vi "saltos.vi"(6 "Comienza Saltos":bool=TRUE, 8 "Nombre Imagen":string="foto", 9 "Path":path, 10 "Parametros de Saltos":T1={"Numero de Saltos"=6, "Paso del Salto (Hz)"=100.0, "Tiempo de estabilizacion (s)"=1.0, "Frequencia de estabilizacion (Hz)"=2000.0, "Tiempo de rampa ON (s)"=5.0, "Tiempo de rampa OFF (s)"=1.0}, 11 "Numero Ultimo Experimento":i32) -> (0 "Tomando Saltos":bool=TRUE, 1 "Estable":bool=TRUE, 2 "appended path":path, 3 "Freq Output":dbl, 4 "Numero Actual Experimento":i32, 5 "Captura Imagen":bool=TRUE)   [LabVIEW 2010]
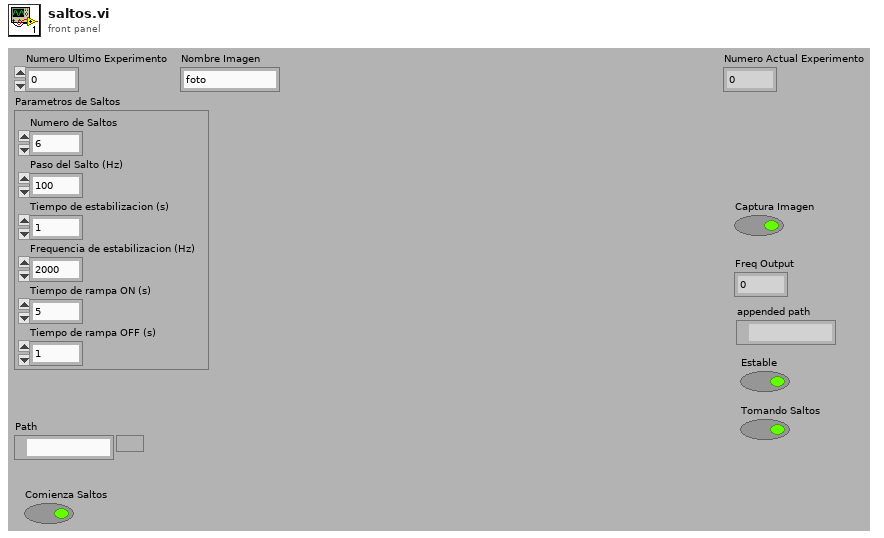
[diagram p1: front panel]
types:
  T1 = cluster{"Numero de Saltos":i32, "Paso del Salto (Hz)":dbl, "Tiempo de estabilizacion (s)":dbl, "Frequencia de estabilizacion (Hz)":dbl, "Tiempo de rampa ON (s)":dbl, "Tiempo de rampa OFF (s)":dbl}
  T2 = enum16{"Rampa ON", "Saltos", "Espera", "Toma Imagen", "Estable", "Rampa OFF", "Espera Estable"}
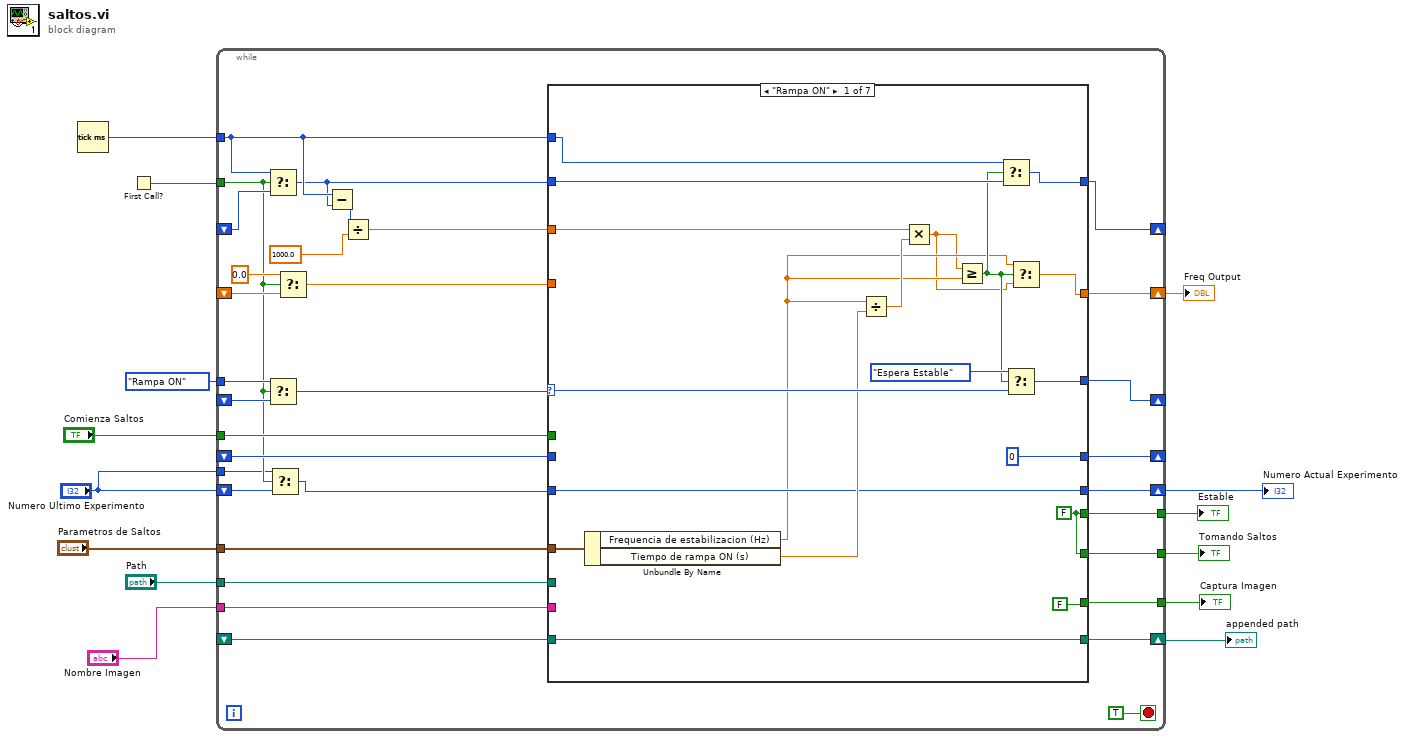
[diagram p0: block diagram]
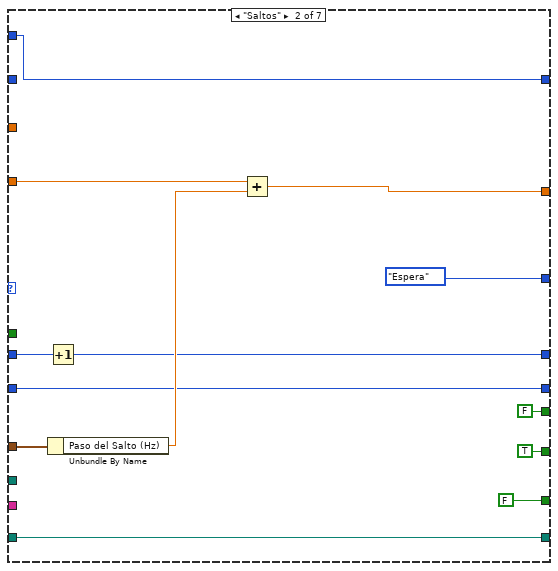
[diagram p2: hidden frame]
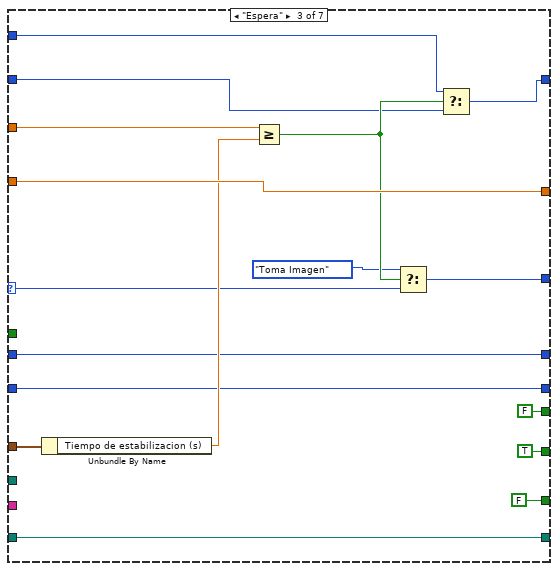
[diagram p3: hidden frame]
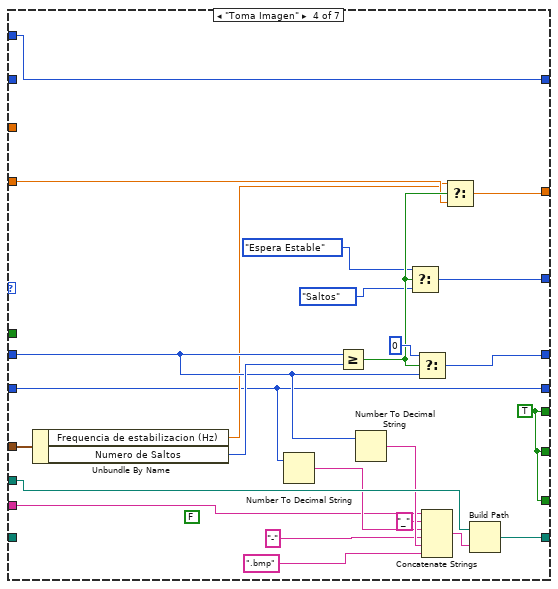
[diagram p4: hidden frame]
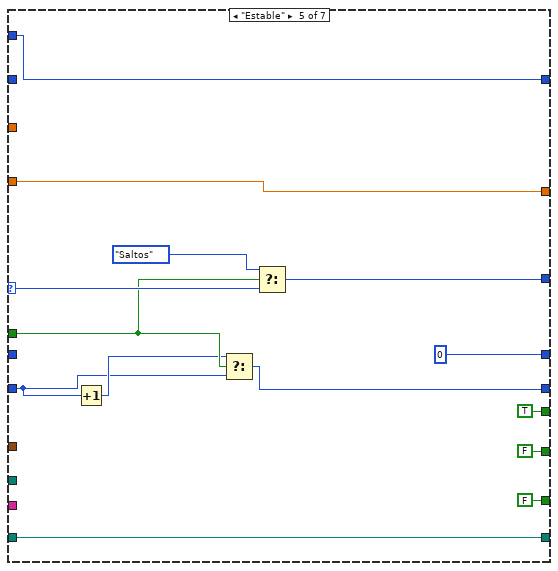
[diagram p5: hidden frame]
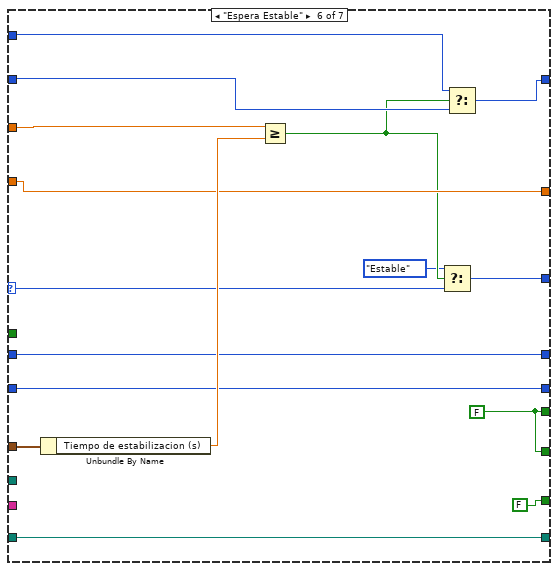
[diagram p6: hidden frame]
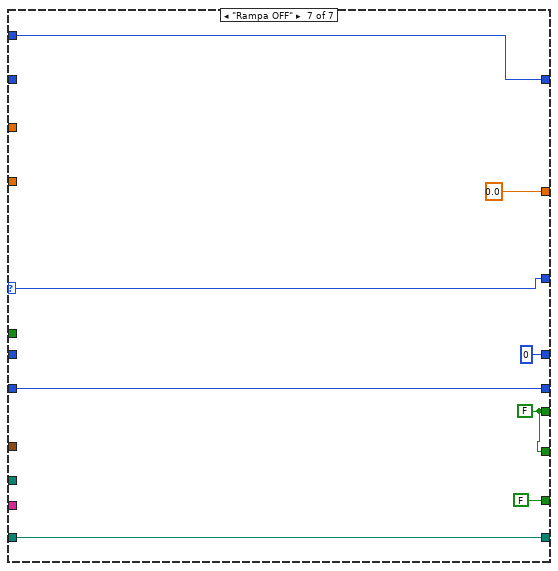
[diagram p7: hidden frame]
diagram:
  n1 = Tick Count (ms)() -> (millisecond timer value=w8:u32)
  n2 = First Call?() -> (First Call?: T/F=w14:bool)
  n3 = while {
    tunnel: w14 -> [w21]
    tunnel: w8 -> [w36]
    shift-right: [w45] -> _
    shift-left: _ -> [w28]
    tunnel: T2."Rampa ON" -> [w41]
    shift-right: [w39] -> _
    shift-left: _ -> [w38]
    tunnel: "Parametros de Saltos" -> [w32]
    tunnel: "Comienza Saltos" -> [w35]
    shift-right: [w34] -> _
    shift-left: _ -> [w33]
    shift-right: [w37] -> w12
    shift-left: _ -> [w31]
    tunnel: "Path" -> [w27]
    shift-right: [w25] -> w5
    shift-left: _ -> [w24]
    tunnel: [w23] -> w7
    tunnel: [w22] -> w6
    tunnel: "Numero Ultimo Experimento" -> [w20]
    shift-right: [w19] -> w4
    shift-left: "Numero Ultimo Experimento" -> [w18]
    tunnel: [w16] -> w3
    tunnel: "Nombre Imagen" -> [w15]
    stop <- TRUE stop-if-true
    n4 = Select(t=w36, s=w21, f=w28) -> (s? t:f=w26:u32)
    n5 = Select(t=w41, s=w21, f=w38) -> (s? t:f=w40:T2)
    n6 = Select(t=w20, s=w21, f=w18) -> (s? t:f=w17:i32)
    n7 = Select(t=0.0, s=w21, f=w31) -> (s? t:f=w29:dbl)
    n8 = Subtract(x=w36, y=w26) -> (x-y=w44:u32)
    n9 = Divide(x=w44, y=1000.0) -> (x/y=w42:dbl)
    n10 = case shown="\"Rampa ON\"" w40 {
      selector: w40 -> [w63 _ w90 _ w133 w141 w153]
      tunnel: [w57 w72 w88 w119 w129 w144 w157] -> w45
      tunnel: w26 -> [w58 _ w85 _ _ w148 _]
      tunnel: w42 -> [w65 _ w93 _ _ w149 _]
      tunnel: [w62 T2."Espera" w91 w116 w132 w140 w153] -> w39
      tunnel: [w47 w73 w95 w107 w130 w143 0.0 ("t")] -> w37
      tunnel: w36 -> [w56 w72 w86 w119 w129 w147 w157]
      tunnel: w35 -> [_ _ _ _ w124 _ _]
      tunnel: [0 w74 w89 w115 0 w138 u32 0 ("t")] -> w34
      tunnel: w29 -> [_ w78 w95 w108 w130 w143 _]
      tunnel: w33 -> [_ w75 w89 w112 _ w138 _]
      tunnel: w32 -> [w61 w77 w94 w118 _ w146 _]
      tunnel: w27 -> [_ _ _ w113 _ _ _]
      tunnel: [w55 w71 w84 w104 w128 w137 w154] -> w25
      tunnel: w24 -> [w55 w71 w84 _ w128 w137 w154]
      tunnel: [w53 FALSE FALSE w98 TRUE w136 w152] -> w23
      tunnel: [w53 TRUE TRUE w98 FALSE w136 w152] -> w22
      tunnel: w17 -> [w52 w67 w80 w100 w122 w135 w151]
      tunnel: [w52 w67 w80 w100 w121 w135 w151] -> w19
      tunnel: [FALSE FALSE FALSE w98 FALSE FALSE FALSE] -> w16
      tunnel: w15 -> [_ _ _ w97 _ _ _]
      frame "Rampa ON" {
        w53 = FALSE
        n11 = Unbundle By Name(w61) -> ("Frequencia de estabilizacion (Hz)"=w49:dbl, "Tiempo de rampa ON (s)"=w60:dbl)
        n12 = Divide(x=w49, y=w60) -> (x/y=w64:dbl)
        n13 = Multiply(x=w65, y=w64) -> (x*y=w48:dbl)
        n14 = Greater Or Equal?(x=w48, y=w49) -> (x >= y?=w50:bool)
        n15 = Select(t=w56, s=w50, f=w58) -> (s? t:f=w57:u32)
        n16 = Select(t=T2."Espera Estable", s=w50, f=w63) -> (s? t:f=w62:T2)
        n17 = Select(t=w49, s=w50, f=w48) -> (s? t:f=w47:dbl)
      }
      frame "Saltos" {
        n18 = Increment(x=w75) -> (x+1=w74:u32)
        n19 = Unbundle By Name(w77) -> ("Paso del Salto (Hz)"=w76:dbl)
        n20 = Add(x=w78, y=w76) -> (x+y=w73:dbl)
      }
      frame "Espera" {
        n21 = Unbundle By Name(w94) -> ("Tiempo de estabilizacion (s)"=w92:dbl)
        n22 = Greater Or Equal?(x=w93, y=w92) -> (x >= y?=w87:bool)
        n23 = Select(t=T2."Toma Imagen", s=w87, f=w90) -> (s? t:f=w91:T2)
        n24 = Select(t=w86, s=w87, f=w85) -> (s? t:f=w88:u32)
      }
      frame "Toma Imagen" {
        w98 = TRUE
        (unwired) FALSE ("Compress? (N)")
        n25 = Unbundle By Name(w118) -> ("Frequencia de estabilizacion (Hz)"=w105:dbl, "Numero de Saltos"=w117:i32)
        n26 = Number To Decimal String(number=w100) -> (decimal integer string=w101:string)  [unwired: 1 in]
        n27 = Greater Or Equal?(x=w112, y=w117) -> (x >= y?=w109:bool)
        n28 = Number To Decimal String(number=w112) -> (decimal integer string=w111:string)  [unwired: 1 in]
        n29 = Select(t=T2."Espera Estable", s=w109, f=T2."Saltos") -> (s? t:f=w116:T2)
        n30 = Select(t=u32 0, s=w109, f=w112) -> (s? t:f=w115:u32)
        n31 = Concatenate Strings(w97, "_" ("string"), w101, "-" ("string"), w111, ".bmp" ("string")) -> (w110:string)
        n32 = Select(t=w105, s=w109, f=w108) -> (s? t:f=w107:dbl)
        n33 = Build Path(base path=w113, name or relative path=w110) -> (appended path=w104:path)
      }
      frame "Estable" {
        n34 = Increment(x=w122) -> (x+1=w123:i32)
        n35 = Select(t=w123, s=w124, f=w122) -> (s? t:f=w121:i32)
        n36 = Select(t=T2."Saltos", s=w124, f=w133) -> (s? t:f=w132:T2)
      }
      frame "Espera Estable" {
        w136 = FALSE
        n37 = Unbundle By Name(w146) -> ("Tiempo de estabilizacion (s)"=w145:dbl)
        n38 = Greater Or Equal?(x=w149, y=w145) -> (x >= y?=w142:bool)
        n39 = Select(t=T2."Estable", s=w142, f=w141) -> (s? t:f=w140:T2)
        n40 = Select(t=w147, s=w142, f=w148) -> (s? t:f=w144:u32)
      }
      frame "Rampa OFF" {
        w152 = FALSE
      }
    }
  }
  "Freq Output" <- w12
  "appended path" <- w5
  "Tomando Saltos" <- w6
  "Estable" <- w7
  "Captura Imagen" <- w3
  "Numero Actual Experimento" <- w4
